vi "OE2011&OE2021_Query PLL&Overload.vi"(0 "VISA resource name":refnum<visa-resource-name>, 5 "Connection ID in":refnum<k5>, 7 "Timeout":u32=1000, 9 "Remote Mode":u16(ring) items=["USB", "RS232", "GPIB", "Ethernet"], 11 "Error in (no error)":errorcluster caption="error out（no error）") -> (4 "VISA resource  out":refnum<visa-resource-name>, 6 "Connection ID out":refnum<k5>, 8 "OE2011&OE2021_\nQuery PLL&Overload":T1, 10 "Output String":string, 15 "Error out":errorcluster caption="error out")   [LabVIEW 2011]
panel:
  in  "Osc Channel":u16(ring)=1 items=["OSC1"=1, "OSC2"=2]
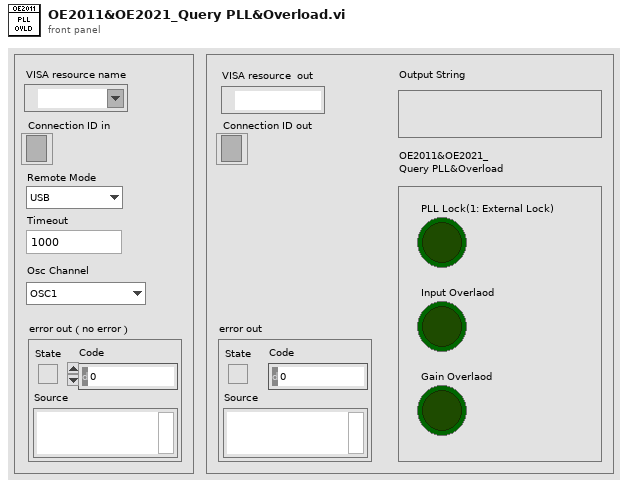
[diagram p1: front panel]
types:
  T1 = cluster{"PLL Lock(1: External Lock)":bool, "Input Overlaod":bool, "Gain Overlaod":bool}
  T2 = enum16{"ISRC", "IGND", "ICPL", "ILIN", "PHAS", "FMOD", "RSLP", "FREQ", "SWPT", "SLLM", "SULM", "SSLL", "SSLG", "STLM", "SWRM", "IRNG", "SENS", "RMOD", "OFLT", "OFSL", "SYNC", "DMOD", "HARM", "DARB", "SWVT", "SLVL", "SVLL", "SVUL", "SVSL", "SVSG", "SVTM", "SVRM", "RALL", "SNAP", "OUTP", "OAUX", "COUT", "CAUX", "COFP", "CEXP", "FPOP", "OEXP", "*IDN", "*RST", "OVLD", "INOV", "GNOV", "*PLL", "SSET", "RSET", "AGAN", "APHS", "ARSV", "ASCL", "EQCD", "EQCS", "SPED", "SRAT", "SLEN", "SSLE", "STRG", "SPRM", "STRD", "PAUS", "REST", "SPTS", "TRCA", "TEMP", "RSTU", "IHNZ", "DEQU", "SADD", "ARNG", "CSPE", "ISRCD", "IGNDD", "ICPLD", "ILIND", "PHASD", "FMODD", "RSLPD", "FREQD", "SWPTD", "SLLMD", "SULMD", "SSLLD", "SSLGD", "STLMD", "SWRMD", "SENSD", "RMODD", "OFLTD", "OFSLD", "SYNCD", "HARMD", "EQCDD", "EQCSD", "SNAPD", "OUTPD", "SWVTD", "SLVLD", "SVLLD", "SVULD", "SVSLD", "SVSGD", "SVTMD", "SVRMD", "SVDCD", "ARSVD", "AGAND", "APHSD", "ASCLD", "FPOPD", "CAUXD", "OEXPD", "SPEDD", "SRATD", "SLEND", "SSLED", "STRGD", "SPRMD", "STRDD", "PAUSD", "RESTD", "SPTSD", "TRCAD", "*IDND", "*RSTD", "INOVD", "GNOVD", "*PLLD", "SSETD", "RSETD"}
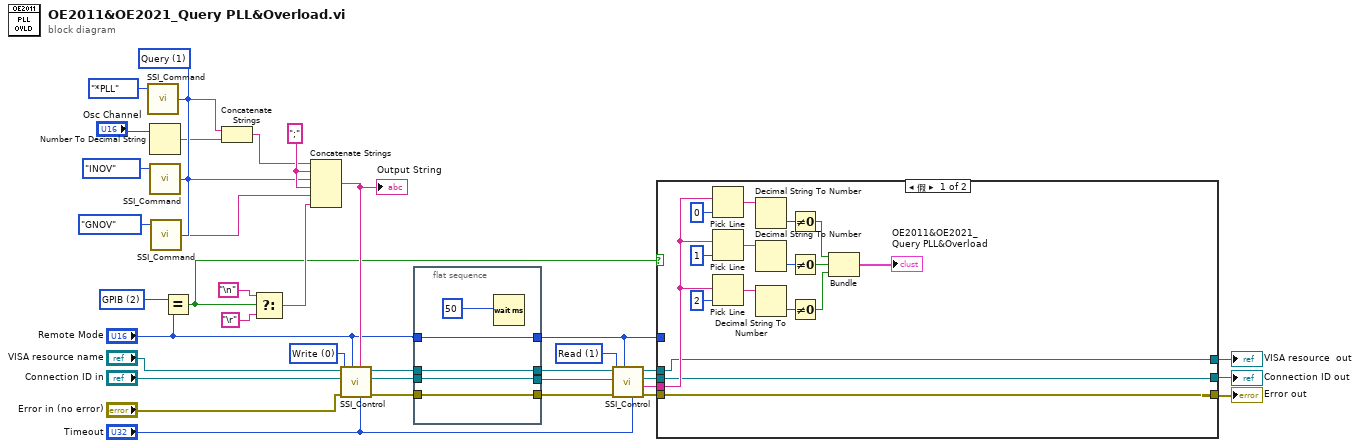
[diagram p0: block diagram]
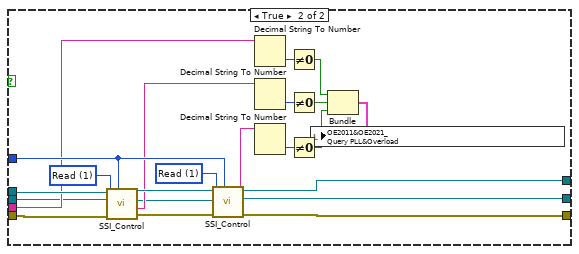
[diagram p2: hidden frame]
diagram:
  w22 = u16 2 items=["USB", "RS232", "GPIB", "Ethernet"] ("Remote Mode")
  w26 = ";"
  w30 = u16 1 items=["Write", "Read"] ("Control")
  w28 = u16 1 items=["Set", "Query"] ("Opera")
  w38 = u16 0 items=["Write", "Read"] ("Control")
  n1 = call "SSI_Command.vi"("Opera"=w28, "Command Type"=T2."*PLL") -> ("Output string"=w4:string)  [unwired: 2 in]
  n2 = Number To Decimal String(number="Osc Channel") -> (decimal integer string=w6:string)  [unwired: 1 in]
  n3 = call "SSI_Command.vi"("Opera"=w28, "Command Type"=T2."INOV") -> ("Output string"=w8:string)  [unwired: 2 in]
  n4 = call "SSI_Command.vi"("Opera"=w28, "Command Type"=T2."GNOV") -> ("Output string"=w7:string)  [unwired: 2 in]
  n5 = Equal?(x=w22, y="Remote Mode") -> (x = y?=w13:bool)
  n6 = Concatenate Strings(w4, w6) -> (w3:string)
  n7 = Select(t="\n", s=w13, f="\r") -> (s? t:f=w19:string)
  n8 = Concatenate Strings(w3, w26, w8, w26, w7, w19) -> (w31:string)
  "Output String" <- w31
  n9 = call "SSI_Control.vi"("Tineout"="Timeout", "Write Buffer"=w31, "Remote Mode"="Remote Mode", "Error in (no error)"="Error in (no error)", "Control"=w38, "Connection ID in"="Connection ID in", "VISA resource name"="VISA resource name") -> ("Error out"=w36:errorcluster, "Connection ID out"=w24:refnum<k5>, "VISA resource  out"=w35:refnum<visa-resource-name>)  [unwired: 1 in, 1 out]
  n10 = flat-sequence {
    tunnel: [w43] -> w34
    tunnel: w36 -> [w43]
    tunnel: [w42] -> w33
    tunnel: w35 -> [w42]
    tunnel: "Remote Mode" -> [w41]
    tunnel: [w41] -> w14
    tunnel: w24 -> [w40]
    tunnel: [w40] -> w23
    frame #0 {
      n11 = Wait (ms)(milliseconds to wait=u32 50 ("等待时间（毫秒）")) -> ()  [unwired: 1 out]
    }
  }
  n12 = call "SSI_Control.vi"("Tineout"="Timeout", "Remote Mode"=w14, "Error in (no error)"=w34, "Control"=w30, "Connection ID in"=w23, "VISA resource name"=w33) -> ("Error out"=w18:errorcluster, "Read Buffer"=w27:string, "Connection ID out"=w2:refnum<k5>, "VISA resource  out"=w16:refnum<visa-resource-name>)  [unwired: 2 in]
  n13 = case shown="假" w13 {
    tunnel: w27 -> [w52 w67]
    tunnel: w18 -> [w46 w80]
    tunnel: [w46 w74] -> w17
    tunnel: w16 -> [w45 w81]
    tunnel: [w45 w75] -> w15
    tunnel: w14 -> [_ w76]
    tunnel: w2 -> [w44 w63]
    tunnel: [w44 w61] -> w1
    frame False {
      n14 = Pick Line(multi-line string=w52, line index=0 ("行索引")) -> (output string=w58:string)  [unwired: 1 in]
      n15 = Pick Line(multi-line string=w52, line index=1 ("行索引")) -> (output string=w59:string)  [unwired: 1 in]
      n16 = Pick Line(multi-line string=w52, line index=2 ("行索引")) -> (output string=w54:string)  [unwired: 1 in]
      n17 = Decimal String To Number(string=w58) -> (number=w47:i32)  [unwired: 2 in, 1 out]
      n18 = Decimal String To Number(string=w59) -> (number=w48:i32)  [unwired: 2 in, 1 out]
      n19 = Decimal String To Number(string=w54) -> (number=w49:i32)  [unwired: 2 in, 1 out]
      n20 = Not Equal To 0?(x=w47) -> (x != 0?=w57:bool)
      n21 = Not Equal To 0?(x=w48) -> (x != 0?=w60:bool)
      n22 = Not Equal To 0?(x=w49) -> (x != 0?=w51:bool)
      n23 = Bundle(w57, w60, w51) -> (→"OE2011&OE2021_\nQuery PLL&Overload":cluster{bool, bool, bool})  [unwired: 1 in]
    }
    frame True {
      w79 = u16 1 items=["Write", "Read"] ("Control")
      w82 = u16 1 items=["Write", "Read"] ("Control")
      n24 = call "SSI_Control.vi"("Remote Mode"=w76, "Error in (no error)"=w80, "Control"=w82, "Connection ID in"=w63, "VISA resource name"=w81) -> ("Error out"=w77:errorcluster, "Read Buffer"=w66:string, "Connection ID out"=w62:refnum<k5>, "VISA resource  out"=w78:refnum<visa-resource-name>)  [unwired: 3 in]
      n25 = call "SSI_Control.vi"("Remote Mode"=w76, "Error in (no error)"=w77, "Control"=w79, "Connection ID in"=w62, "VISA resource name"=w78) -> ("Error out"=w74:errorcluster, "Read Buffer"=w65:string, "Connection ID out"=w61:refnum<k5>, "VISA resource  out"=w75:refnum<visa-resource-name>)  [unwired: 3 in]
      n26 = Decimal String To Number(string=w67) -> (number=w68:i32)  [unwired: 2 in, 1 out]
      n27 = Decimal String To Number(string=w66) -> (number=w69:i32)  [unwired: 2 in, 1 out]
      n28 = Decimal String To Number(string=w65) -> (number=w70:i32)  [unwired: 2 in, 1 out]
      n29 = Not Equal To 0?(x=w68) -> (x != 0?=w72:bool)
      n30 = Not Equal To 0?(x=w69) -> (x != 0?=w73:bool)
      n31 = Not Equal To 0?(x=w70) -> (x != 0?=w71:bool)
      n32 = Bundle(w72, w73, w71) -> (w64:cluster{bool, bool, bool})  [unwired: 1 in]
      n33 = local write "OE2011&OE2021_\nQuery PLL&Overload"(w64) -> ()
    }
  }
  "Error out" <- w17
  "VISA resource  out" <- w15
  "Connection ID out" <- w1
